vi "Serial.vi"() -> ()   [LabVIEW 2016]
uses:
  <vilib>/Instr/_visa.llb/VISA Configure Serial Port (Instr).vi
panel:
  in  "Stop Button":bool
  out "read buffer":string
  in  "write buffer":string
  in  "Cluster":T1={"VISA resource name"="", "baud rate (9600)"=9600, "data bits (8)"=8, "error in (no error)"={"status"=FALSE, "code"=0, "source"=""}, "parity (0:none)"=0, "stop bits (10: 1 bit)"=10, "flow control (0:none)"=0} {"flow control (0:none)" items=["None", "XON/XOFF", "RTS/CTS", "XON/XOFF & RTS/CTS", "DTR/DSR", "XON/XOFF & DTR/DSR"]; "stop bits (10: 1 bit)" items=["1.0"=10, "1.5"=15, "2.0"=20]; "parity (0:none)" items=["None", "Odd", "Even", "Mark", "Space"]; "data bits (8)" min=5 max=8 step=1}
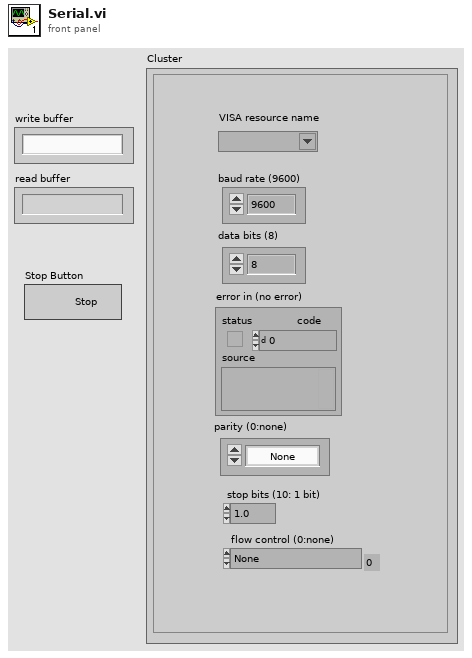
[diagram p1: front panel]
types:
  T1 = cluster{"VISA resource name":refnum<visa-resource-name>, "baud rate (9600)":u32, "data bits (8)":u16, "error in (no error)":errorcluster, "parity (0:none)":u16, "stop bits (10: 1 bit)":u16, "flow control (0:none)":u16}
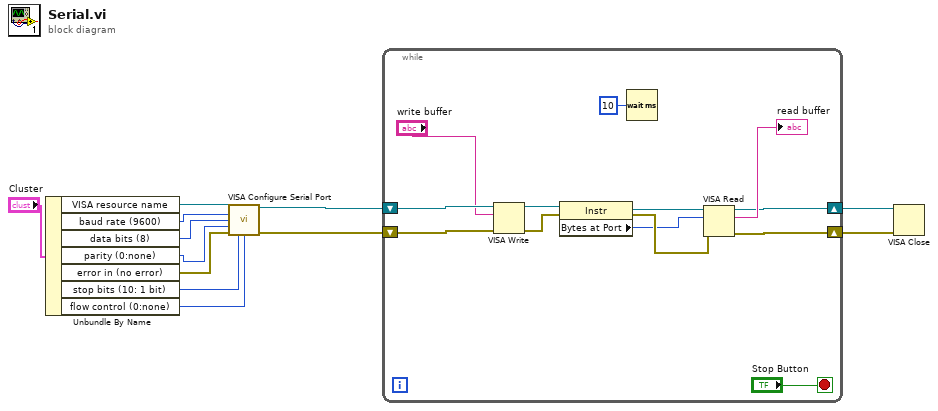
[diagram p0: block diagram]
diagram:
  n1 = Unbundle By Name("Cluster") -> ("VISA resource name"=w7:refnum<visa-resource-name>, "baud rate (9600)"=w8:u32, "data bits (8)"=w9:u16, "parity (0:none)"=w10:u16, "error in (no error)"=w11:errorcluster, "stop bits (10: 1 bit)"=w4:u16, "flow control (0:none)"=w3:u16)
  n2 = call-poly "VISA Configure Serial Port"("VISA resource name"=w7, "baud rate (9600)"=w8, "data bits (8)"=w9, "parity (0:none)"=w10, "error in (no error)"=w11, "stop bits (10: 1 bit)"=w4, "flow control (0:none)"=w3) -> ("VISA resource name out"=w6:refnum<visa-resource-name>, "error out"=w5:errorcluster)  [unwired: 7 in]
  n3 = while {
    shift-right: [w21] -> w2
    shift-left: w6 -> [w25]
    shift-right: [w20] -> w1
    shift-left: w5 -> [w24]
    stop <- "Stop Button" stop-if-true
    n4 = VISA Write(VISA resource name=w25, write buffer="write buffer", error in (no error)=w24) -> (VISA resource name out=w19:refnum<visa-resource-name>, error out=w18:errorcluster)  [unwired: 1 out]
    n5 = property class="Instr"(reference=w19, error in=w18) -> (reference out=w17:refnum<visa-resource-name>, error out=w16:errorcluster, "Bytes at Port"=w15:u32)
    n6 = Wait (ms)(milliseconds to wait=u32 10) -> ()  [unwired: 1 out]
    n7 = VISA Read(VISA resource name=w17, byte count=w15, error in (no error)=w16) -> (VISA resource name out=w21:refnum<visa-resource-name>, read buffer=→"read buffer":string, error out=w20:errorcluster)  [unwired: 1 out]
  }
  n8 = VISA Close(VISA resource name=w2, error in (no error)=w1) -> ()  [unwired: 1 out]
